vi "JSON to LVObject - LVClass Serializer - Is Passed to Serializable Class.vi"() -> ()   [LabVIEW 2017, in "JSON Serializable Serializer Tests.lvlib"]
uses:
  JSON Serializable Serializer Tests.lvlib
  JSON Serializable Serializer/JSON Serializable Serializer.lvclass
  Mock JSON Serializable/Mock JSON Serializable.lvclass/Mock JSON Serializable.ctl
  <vilib>/addons/_JKI Toolkits/Caraya/classes/Assert/Assert Equal Value and Type_Variant.vi
  <vilib>/addons/_JKI Toolkits/Caraya/classes/Test/Test.lvclass
  <vilib>/addons/_JKI Toolkits/Caraya/classes/Assert/Assert.lvclass
  Mock JSON Serializable/Mock JSON Serializable.lvclass
panel:
  out "error out":errorcluster
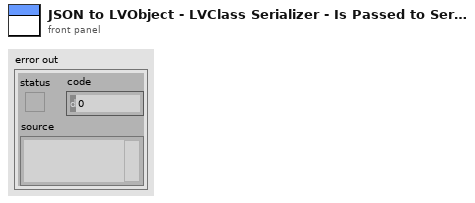
[diagram p1: front panel]
types:
  T1 = cluster{"LVClass Serializer":refnum<class "JSONtext LVClass Serializer.lvclass">, "<JSON>":string, "error in (no error)":errorcluster}
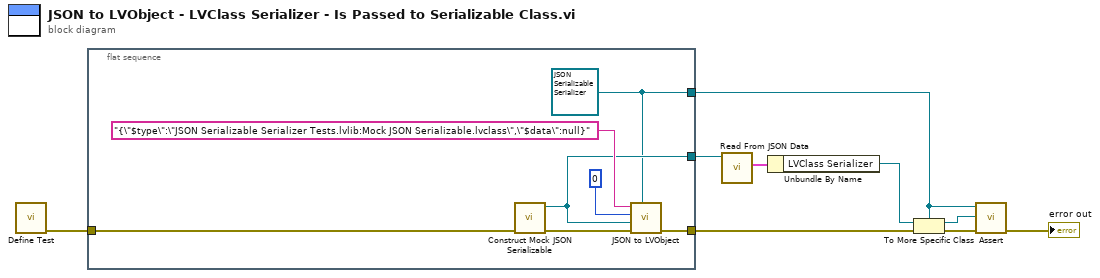
[diagram p0: block diagram]
diagram:
  n1 = call <vilib>:"Define Test.vi"() -> ("error out"=w9:errorcluster)  [unwired: 11 in]
  n2 = flat-sequence {
    tunnel: [w15] -> w7
    tunnel: w9 -> [w12]
    tunnel: [w11] -> w6
    tunnel: [w10] -> w1
    frame #0 {
      w10 = refnum<class "JSON Serializable Serializer.lvclass"> refnum ("JSON Serializer.lvclass")
      n3 = call "Construct Mock JSON Serializable.vi"("error in (no error)"=w12) -> ("error out"=w13:errorcluster, "Mock JSON Serializable"=w11:refnum<class "Mock JSON Serializable.lvclass">)  [unwired: 9 in]
      n4 = call-dynamic "JSON to LVObject.vi"("JSON Serializable Serializer in"=w10, "error in (no error)"=w13, "Object Type"=w11, "Offset"=0, "JSON"="{\"$type\":\"JSON Serializable Serializer Tests.lvlib:Mock JSON Serializable.lvclass\",\"$data\":null}") -> ("error out"=w15:errorcluster)  [unwired: 5 in, 1 out]
    }
  }
  n5 = call "Read From JSON Data.vi"("Mock JSON Serializable in"=w6) -> ("From JSON Data"=w5:T1)  [unwired: 9 in, 1 out]
  n6 = Unbundle By Name(w5) -> ("LVClass Serializer"=w3:refnum<class "JSONtext LVClass Serializer.lvclass">)
  n7 = To More Specific Class(target class=w1, reference=w3, error in=w7) -> (specific class reference=w2:refnum<class "JSON Serializable Serializer.lvclass">, error out=w4:errorcluster)
  n8 = call-poly <vilib>:"Assert.vi"("error in (no error)"=w4, "Y"=w2, "X"=w1) -> ("error out"=→"error out":errorcluster)  [unwired: 8 in]
